vi "[Global]CalTemp.vi"() -> ()   [LabVIEW 2019]
panel:
  in  "CalTemp":cluster{"Script Name":string, "CalImage":T1}[](array[cluster])
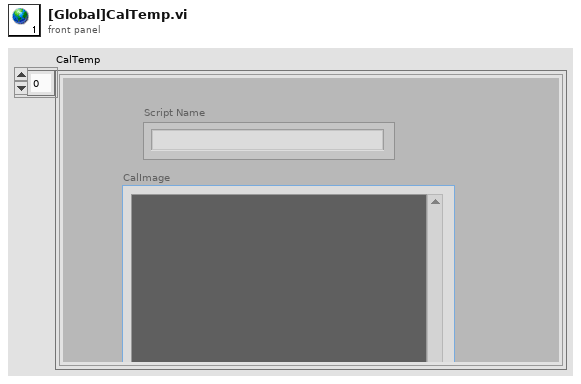
[diagram p1: front panel]
types:
  T1 = typedef "IMAQ Image.ctl" = refnum<image>
diagram:
